vi "Set Tracking Test Settings.vi"(10 "Tracking Test Settings":T1 {"Sample Time (s)" format="%.4f"; "Process Time (s)" format="%.4f"; "Max Moment (NM)" format="%.4f"; "Max Force Error (N)" format="%.4f"}, 11 "Model in":refnum<class "Model.lvclass">) -> (3 "Model out":refnum<class "Model.lvclass">)   [LabVIEW 2016, in "Model.lvclass"]
uses:
  Model.lvclass
  Typedefs/TrackingTestSettings.ctl
  Model.lvclass/Model.ctl
  Typedefs/FAMT Typedefs.lvlib
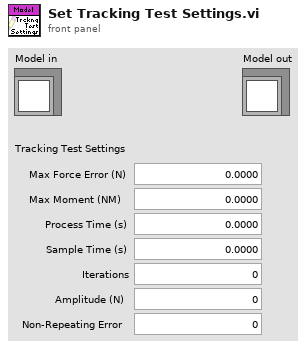
[diagram p1: front panel]
types:
  T1 = typedef "FAMT Typedefs.lvlib/TrackingTestSettings.ctl" = cluster{"Max Force Error (N)":dbl, "Max Moment (NM)":dbl, "Process Time (s)":dbl, "Sample Time (s)":dbl, "Iterations":i32, "Amplitude (N)":dbl, "Non-Repeating Error":dbl}
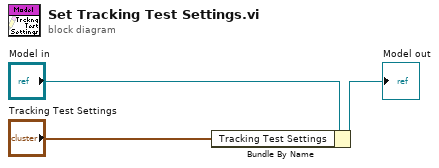
[diagram p0: block diagram]
diagram:
  n1 = Bundle By Name(cluster="Model in", "Tracking Test Settings"="Tracking Test Settings") -> (→"Model out":refnum<class "Model.lvclass">)
